vi "datatypes.vi"() -> ()   [LabVIEW 2021]
panel:
  out "Floating Point 2":dbl
  out "Integer 2":i64
  out "String":string
  in  "Floating Point":dbl
  in  "Integer":i64
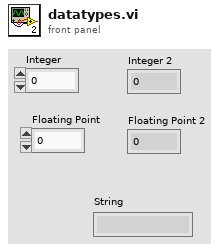
[diagram p1: front panel]
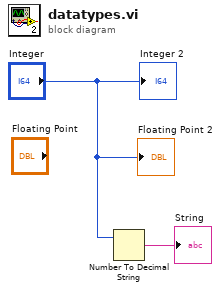
[diagram p0: block diagram]
diagram:
  n1 = Number To Decimal String(number="Integer") -> (decimal integer string=→"String":string)  [unwired: 1 in]
  "Integer 2" <- "Integer"
  "Floating Point 2" <- "Integer"
